vi "VI Tree.vi"   [LabVIEW 2015, in "Global FIA milliGAT.lvlib"]
doc: "This is the instrument driver for the <INSTRUMENT NAME>. The VI Tree displays all the user-callable VIs of the instrument driver in an organized table."
uses:
  Global FIA milliGAT.lvlib
  Action-Status/Start Flow (Specified Volume).vi
  Action-Status/Start Flow (Continuous).vi
panel:
  # "(c) 2014 <Enter Company Name Here>.  ALL RIGHTS RESERVED."
  # "SEE DIAGRAM\nFOR VI TREE."
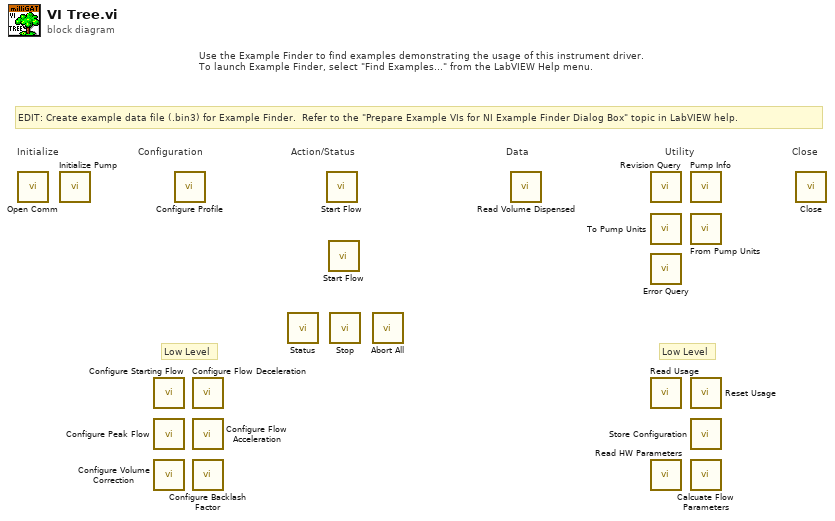
[diagram p0: block diagram]
diagram:
  # "Low Level"
  # "Low Level"
  # "EDIT: Create example data file (.bin3) for Example Finder.  Refer to the \"Prepare Example VIs for NI Example Finder Dialog Box\" topic in LabVIEW help."
  # "Use the Example Finder to find examples demonstrating the usage of this instrument driver.\nTo launch Example Finder, select \"Find Examples...\" from the LabVIEW Help menu."
  # "Configuration"
  # "Utility"
  # "Data"
  # "Action/Status"
  # "Close"
  # "Initialize"
  n1 = call "Open Comm.vi"() -> ()  [unwired: 10 in, 2 out]
  n2 = call "Initialize Pump.vi"() -> ()  [unwired: 10 in, 2 out]
  n3 = call "Configure Starting Flow.vi"() -> ()  [unwired: 10 in, 2 out]
  n4 = call "Configure Peak Flow.vi"() -> ()  [unwired: 10 in, 2 out]
  n5 = call "Configure Volume Correction.vi"() -> ()  [unwired: 10 in, 2 out]
  n6 = call "Configure Profile.vi"() -> ()  [unwired: 10 in, 2 out]
  n7 = call "Configure Flow Deceleration.vi"() -> ()  [unwired: 10 in, 2 out]
  n8 = call "Configure Flow Acceleration.vi"() -> ()  [unwired: 10 in, 2 out]
  n9 = call "Configure Backlash Factor.vi"() -> ()  [unwired: 10 in, 2 out]
  n10 = call "Status.vi"() -> ()  [unwired: 9 in, 3 out]
  n11 = call-poly "Start Flow.vi"() -> ()  [unwired: 10 in, 2 out]
  n12 = call-poly "Start Flow.vi"() -> ()  [unwired: 10 in, 2 out]
  n13 = call "Stop.vi"() -> ()  [unwired: 10 in, 2 out]
  n14 = call "Abort All.vi"() -> ()  [unwired: 10 in, 2 out]
  n15 = call "Read Volume Dispensed.vi"() -> ()  [unwired: 9 in, 3 out]
  n16 = call "Revision Query.vi"() -> ()  [unwired: 8 in, 4 out]
  n17 = call "To Pump Units.vi"() -> ()  [unwired: 10 in, 2 out]
  n18 = call "Error Query.vi"() -> ()  [unwired: 9 in, 3 out]
  n19 = call "Read Usage.vi"() -> ()  [unwired: 9 in, 3 out]
  n20 = call "Read HW Parameters.vi"() -> ()  [unwired: 9 in, 3 out]
  n21 = call "Pump Info.vi"() -> ()  [unwired: 8 in, 4 out]
  n22 = call "From Pump Units.vi"() -> ()  [unwired: 10 in, 2 out]
  n23 = call "Reset Usage.vi"() -> ()  [unwired: 10 in, 2 out]
  n24 = call "Store Configuration.vi"() -> ()  [unwired: 10 in, 2 out]
  n25 = call "Calcuate Flow Parameters.vi"() -> ()  [unwired: 9 in, 3 out]
  n26 = call "Close.vi"() -> ()  [unwired: 11 in, 1 out]
